vi "write camera json.vi"(8 "error in (no error)":errorcluster, 11 "Save Image ECHARPE in":refnum<class "Save Image ECHARPE.lvclass">) -> (0 "error out":errorcluster, 3 "Save Image ECHARPE out":refnum<class "Save Image ECHARPE.lvclass">)   [LabVIEW 2018, in "Save Image ECHARPE.lvclass"]
doc: "Prepare the header content to be provided to the Python toolkit\n\nThis function returns a JSON with the information to be written into the image header"
uses:
  Save Image ECHARPE.lvclass
  S4ACS/src/LabVIEW/ECHARPE Cam OpMode/ECHARPE Cam OpMode.lvclass/ECHARPE Cam OpMode.ctl
  S4ACS/src/LabVIEW/Save Image/Save Image.lvclass
  S4ACS/src/LabVIEW/Channel ECHARPE/Channel ECHARPE.lvclass
  S4ACS/src/LabVIEW/Camera Simulated iKon/Camera Simulated iKon.lvclass
  S4ACS/src/LabVIEW/ECHARPE Cam OpMode/ECHARPE Cam OpMode.lvclass
panel:
  in  "prev ikon op mode":cluster{"HIGHCAP":bool}
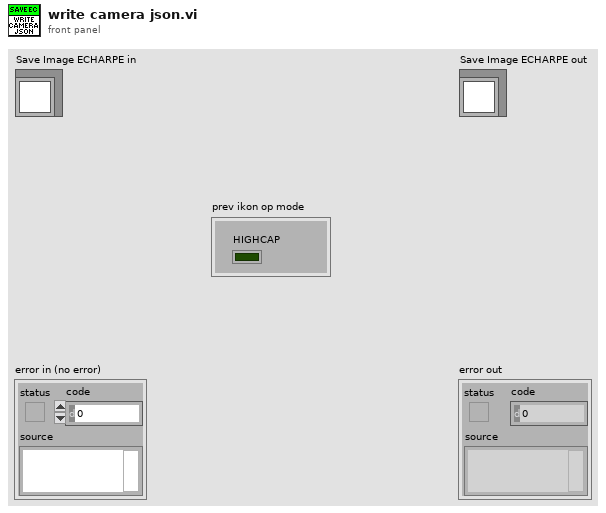
[diagram p1: front panel]
types:
  T1 = cluster{"CCD":string, "GUI":string, "ICS":string, "TCS":string, "FOCUSER":string, "WSTATION":string, "GENERAL KW":string}
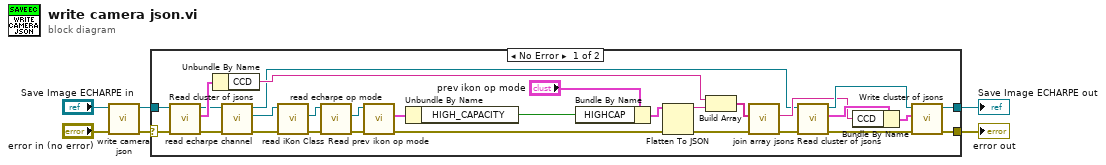
[diagram p0: block diagram]
diagram:
  n1 = call-parent "write camera json.vi"("error in (no error)"="error in (no error)", "Save Image in"="Save Image ECHARPE in") -> ("error out"=w4:errorcluster, "Save Image out"=w2:refnum<class "Save Image ECHARPE.lvclass">)  [unwired: 8 in]
  n2 = case shown="No Error" w4 {
    selector: w4 -> [w23 w37]
    tunnel: [w21 w37] -> w3
    tunnel: w2 -> [w24 w36]
    tunnel: [w22 w36] -> w1
    frame No Error {
      n3 = call-dynamic "Read cluster of jsons.vi"("error in (no error)"=w23, "Save Image in"=w24) -> ("error out"=w20:errorcluster, "cluster of jsons"=w34:T1, "Save Image out"=w19:refnum<class "Save Image ECHARPE.lvclass">)  [unwired: 7 in]
      n4 = Unbundle By Name(w34) -> ("CCD"=w33:string)
      n5 = call "read echarpe channel.vi"("error in (no error)"=w20, "Save Image ECHARPE in"=w19) -> ("error out"=w17:errorcluster, "echarpe channel"=w18:refnum<class "Channel ECHARPE.lvclass">, "Save Image ECHARPE out"=w11:refnum<class "Save Image ECHARPE.lvclass">)  [unwired: 7 in]
      n6 = call "read iKon Class.vi"("error in (no error)"=w17, "SPARC4_Channel in"=w18) -> ("error out"=w15:errorcluster, "Camera Simulated iKon.lvclass"=w16:refnum<class "Camera Simulated iKon.lvclass">)  [unwired: 7 in, 1 out]
      n7 = call "read echarpe op mode.vi"("error in (no error)"=w15, "Camera Simulated iKon in"=w16) -> ("error out"=w13:errorcluster, "ECHARPE Cam OpMode.lvclass"=w14:refnum<class "ECHARPE Cam OpMode.lvclass">)  [unwired: 7 in, 1 out]
      n8 = call "Read prev ikon op mode.vi"("error in (no error)"=w13, "ECHARPE Cam OpMode in"=w14) -> ("error out"=w12:errorcluster, "prev ikon op mode"=w9:cluster{"HIGH_CAPACITY":bool})  [unwired: 7 in, 1 out]
      n9 = Unbundle By Name(w9) -> ("HIGH_CAPACITY"=w8:bool)
      n10 = Bundle By Name(cluster="prev ikon op mode", "HIGHCAP"=w8) -> (w7:cluster{"HIGHCAP":bool})
      n11 = Flatten To JSON(anything=w7, error in (no error)=w12) -> (JSON string=w35:string, 11:w26:errorcluster)  [unwired: 1 in]
      n12 = Build Array(w33, w35) -> (w25:string[])
      n13 = call "join array jsons.vi"("error in (no error)"=w26, "jsons"=w25) -> ("error out"=w27:errorcluster, "concatenated json"=w28:string)  [unwired: 8 in]
      n14 = call-dynamic "Read cluster of jsons.vi"("error in (no error)"=w27, "Save Image in"=w11) -> ("error out"=w32:errorcluster, "cluster of jsons"=w30:T1, "Save Image out"=w31:refnum<class "Save Image ECHARPE.lvclass">)  [unwired: 7 in]
      n15 = Bundle By Name(cluster=w30, "CCD"=w28) -> (w29:T1)
      n16 = call-dynamic "Write cluster of jsons.vi"("error in (no error)"=w32, "cluster of jsons"=w29, "Save Image in"=w31) -> ("error out"=w21:errorcluster, "Save Image out"=w22:refnum<class "Save Image ECHARPE.lvclass">)  [unwired: 7 in]
    }
    frame Error {
    }
  }
  "error out" <- w3
  "Save Image ECHARPE out" <- w1
